vi "Encrypt.vi"(10 "String":string, 11 "iEncryption in":refnum<class "iEncryption.lvclass">) -> (2 "Encrypted String":string)   [LabVIEW 2019, in "User Configuration Manager.lvlib" / "iEncryption.lvclass"]
uses:
  <vilib>/gpm_packages/@cs/user-manager/Source/iEncryption/iEncryption.lvclass
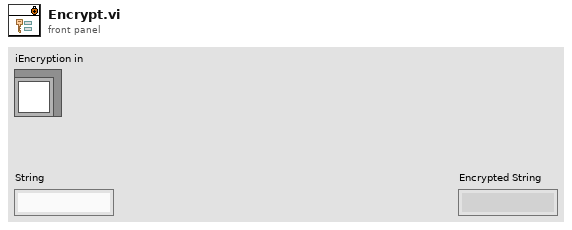
[diagram p1: front panel]
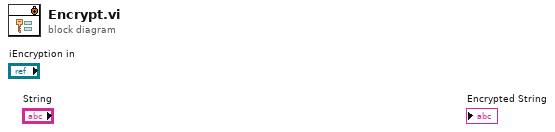
[diagram p0: block diagram]
diagram:
